vi "getGain.vi"(8 "error in (no error)":errorcluster, 11 "Instrument.Lockin in":refnum<class "Instrument.Lockin.lvclass">) -> (0 "error out":errorcluster, 2 "Gain":dbl[](array[numeric]), 3 "Instrument.Lockin out":refnum<class "Instrument.Lockin.lvclass">)   [LabVIEW 2016, in "Instrument.Lockin.lvclass"]
doc: "API to get the AI waveforms.\n\nIf address=\"\", this API reads from localhost\nIf address is remote lockin, you need to add this computer to allowed whitelist on the lockin computer you are trying to access."
uses:
  Instrument.Lockin.lvclass
  Typedefs/Instrument.Lockin.Commands--Enum.ctl
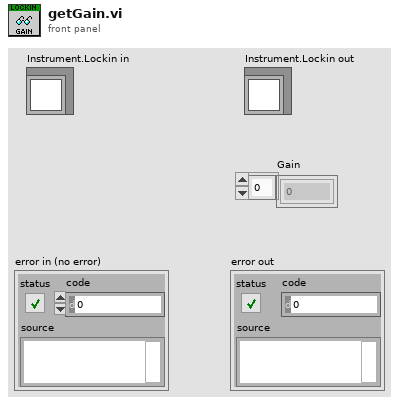
[diagram p1: front panel]
types:
  T1 = typedef "Instrument.Lockin.lvclass/Instrument.Lockin.Commands--Enum.ctl" = enum16{"setAO", "setAO_Amplitude", "setAO_DC", "setAO_Frequency", "setAO_Phase", "setAO_Function", "setAO_I+", "setREF", "setREF_Frequency", "setREF_Phase", "setREF_Filter", "setIVmode", "Reset", "setSampling", "Trigger", "getAO", "getAI", "getResults", "getTrigger", "getIVmode", "getSampling", "getAOconfig", "getREFconfig", "getREF_Filter", "setGain", "getGain", "setAutoSampling", "getAutoSampling", "setSweep", "getStatus", "getSweepResults", "startSweep", "stopSweep"}
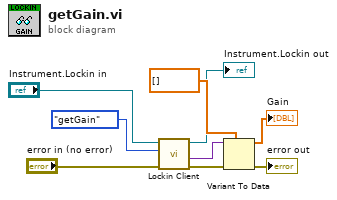
[diagram p0: block diagram]
diagram:
  n1 = call "Lockin Client.vi"("error in (no error)"="error in (no error)", "Command"=Instrument.Lockin.Commands--Enum."getGain", "Instrument.Lockin in"="Instrument.Lockin in") -> ("error out"=w8:errorcluster, "Data out"=w9:variant, "Instrument.Lockin out"=→"Instrument.Lockin out":refnum<class "Instrument.Lockin.lvclass">)  [unwired: 6 in]
  n2 = Variant To Data(error in=w8, type=dbl[] [] ("Gain"), Variant=w9) -> (data=→"Gain":dbl[], error out=→"error out":errorcluster)
